vi "doAction.vi"(8 "error in (no error)":errorcluster, 10 "ContextData":refnum<class "ContextData.lvclass">, 11 "Run in":refnum<class "Welcome.lvclass">) -> (0 "error out":errorcluster, 2 "ContextData Out":refnum<class "ContextData.lvclass">, 3 "Run out":refnum<class "Welcome.lvclass">)   [LabVIEW 2020, in "Welcome.lvclass"]
uses:
  Welcome.lvclass
  ContextData/ContextData.lvclass
  uiControlsMgr/uiControlsMgr.lvclass
  Messages/simonMessages/simonMessages.lvclass
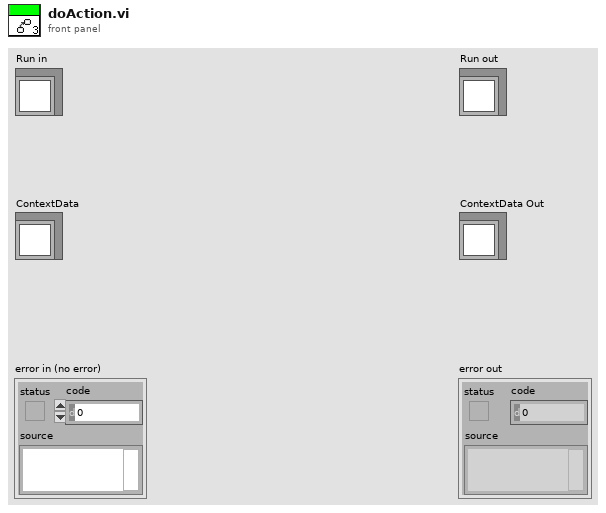
[diagram p1: front panel]
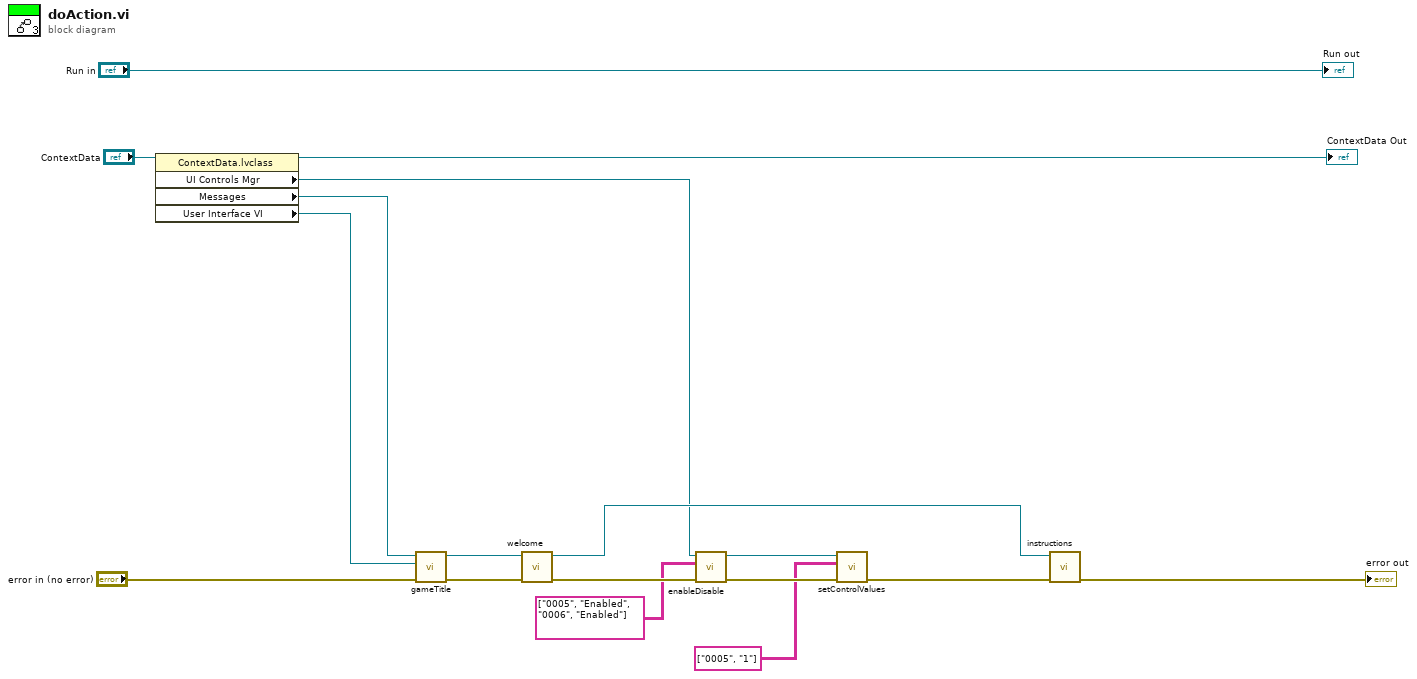
[diagram p0: block diagram]
diagram:
  n1 = property class="ContextData.lvclass"(reference="ContextData") -> (reference out=→"ContextData Out":refnum<class "ContextData.lvclass">, "UI Controls Mgr"=w11:refnum<class "uiControlsMgr.lvclass">, "Messages"=w5:refnum<class "simonMessages.lvclass">, "User Interface VI"=w1:refnum<vi>)  [unwired: 1 in, 1 out]
  n2 = call "gameTitle.vi"("error in (no error)"="error in (no error)", "VI Refnum"=w1, "simonMessages in"=w5) -> ("error out"=w2:errorcluster, "simonMessages out"=w4:refnum<class "simonMessages.lvclass">)  [unwired: 7 in]
  n3 = call "welcome.vi"("error in (no error)"=w2, "simonMessages in"=w4) -> ("error out"=w13:errorcluster, "simonMessages out"=w14:refnum<class "simonMessages.lvclass">)  [unwired: 8 in]
  n4 = call "enableDisable.vi"("error in (no error)"=w13, "Controls - Status"=string[][] [["0005", "Enabled"], ["0006", "Enabled"]], "uiControlsMgr in"=w11) -> ("error out"=w9:errorcluster, "uiControlsMgr out"=w7:refnum<class "uiControlsMgr.lvclass">)  [unwired: 7 in]
  n5 = call "setControlValues.vi"("error in (no error)"=w9, "Controls - Value"=string[][] [["0005", "1"]], "uiControlsMgr in"=w7) -> ("error out"=w8:errorcluster)  [unwired: 7 in, 1 out]
  n6 = call "instructions.vi"("error in (no error)"=w8, "simonMessages in"=w14) -> ("error out"=→"error out":errorcluster)  [unwired: 8 in, 1 out]
  "Run out" <- "Run in"
